vi "read_params.vi"(8 "error in (no error)":errorcluster, 11 "DecisionTreeClassifier in":refnum<class "DecisionTreeClassifier.lvclass">) -> (0 "error out":errorcluster, 2 "params":T1={"criterion"="gini", "splitter"="random", "max_depth"={"max_depth_type"="None", "max_depth_int"=0.0}, "min_samples_split"=2.0, "min_samples_leaf"=1.0, "min_weight_fraction_leaf"=0.0, "max_features"={"max_features_type"="None", "max_features_int"=0.0, "max_features_float"=0.0}, "random_state"=0.0, "max_leaf_nodes"={"max_leaf_nodes_type"="None", "max_leaf_nodes_int"=100.0}, "min_impurity_decrease"=0.0, "class_weight"={"class_weight_type"="None", "class_weight_dict"="{0:1.1, 2:1.5, 2:0.6}"}, "ccp_alpha"=0.0}, 3 "DecisionTreeClassifier out":refnum<class "DecisionTreeClassifier.lvclass">)   [LabVIEW 2020, in "DecisionTreeClassifier.lvclass"]
uses:
  DecisionTreeClassifier.lvclass
  Controls/decision_tree_classifier_params.ctl
  DecisionTreeClassifier.lvclass/DecisionTreeClassifier.ctl
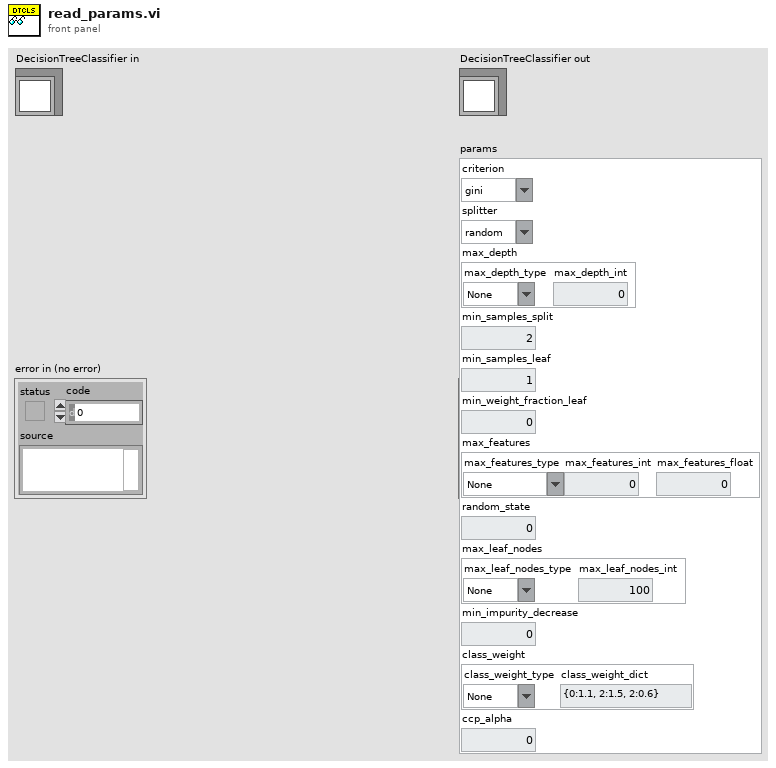
[diagram p1: front panel]
types:
  T1 = typedef "decision_tree_classifier_params.ctl" = cluster{"criterion":string, "splitter":string, "max_depth":cluster{"max_depth_type":string, "max_depth_int":dbl}, "min_samples_split":dbl, "min_samples_leaf":dbl, "min_weight_fraction_leaf":dbl, "max_features":cluster{"max_features_type":string, "max_features_int":dbl, "max_features_float":dbl}, "random_state":dbl, "max_leaf_nodes":cluster{"max_leaf_nodes_type":string, "max_leaf_nodes_int":dbl}, "min_impurity_decrease":dbl, "class_weight":cluster{"class_weight_type":string, "class_weight_dict":string}, "ccp_alpha":dbl}
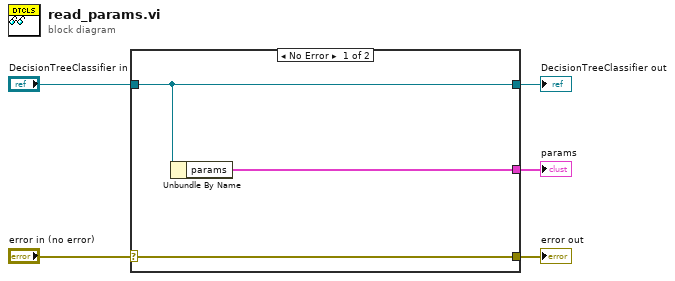
[diagram p0: block diagram]
diagram:
  n1 = case shown="No Error" "error in (no error)" {
    selector: "error in (no error)" -> [w8 w9]
    tunnel: [w8 w9] -> w4
    tunnel: [w7 w10] -> w2
    tunnel: "DecisionTreeClassifier in" -> [w7 w10]
    tunnel: [w6 _] -> w1
    frame No Error {
      n2 = Unbundle By Name(w7) -> ("params"=w6:T1)
    }
    frame Error {
    }
  }
  "error out" <- w4
  "DecisionTreeClassifier out" <- w2
  "params" <- w1
